vi "Rohde & Schwarz VNA Read Number of Ports.vi"(7 "Rohde & Schwarz VNA":T1, 8 "error in (no error)":errorcluster, 11 "VISA Resource Name":refnum<visa-resource-name>) -> (0 "error out":errorcluster, 2 "Number of Ports":i8, 3 "dup VISA Resource Name":refnum<visa-resource-name>)   [LabVIEW 2011]
doc: "This VI for the HP 8753 is used to read the sweep type.\n\n0 LINEAR FREQ\n1 LOG FREQ\n2 LIST FREQ\n3 CW TIME\n4 POWER SWEEP"
uses:
  TypeDefs/Rohde & Schwarz VNA Instrument Info.ctl
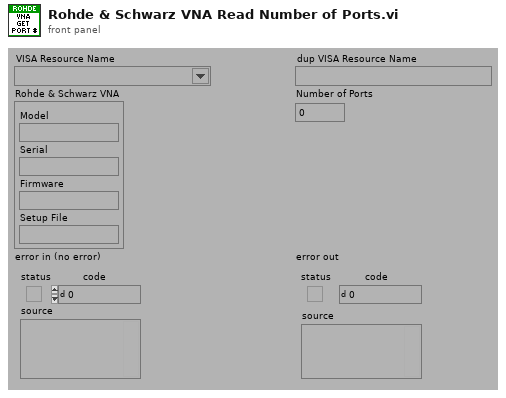
[diagram p1: front panel]
types:
  T1 = typedef "Rohde & Schwarz VNA Instrument Info.ctl" = cluster{"Model":string, "Serial":string, "Firmware":string, "Setup File":string}
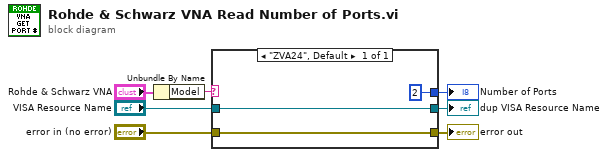
[diagram p0: block diagram]
diagram:
  n1 = Unbundle By Name("Rohde & Schwarz VNA") -> ("Model"=w1:string)
  n2 = case shown="\"ZVA24\", Default" w1 {
    tunnel: "VISA Resource Name" -> [w10]
    tunnel: "error in (no error)" -> [w9]
    tunnel: [w9] -> w6
    tunnel: [i8 2] -> w5
    tunnel: [w10] -> w3
    frame "ZVA24", Default {
    }
  }
  "Number of Ports" <- w5
  "dup VISA Resource Name" <- w3
  "error out" <- w6
